vi "ziExample-Module-SweepUtility.vi"() -> ()   [LabVIEW 2009]
doc: "Control a Zurich instrument device via the LabOne Labview API. \nRequirements: Zurich Instruments MFLI, HF2 or UHFLI \nThis example shows how to start a sweeper module and retrieve data in an interactive vi.\n\n© Zurich Instruments AG, www.zhinst.com"
uses:
  <instrlib>/Zurich Instruments LabOne/Public/Modules/ziTypeModResults.ctl
  <instrlib>/Zurich Instruments LabOne/Public/Data/ziTypePollType.ctl
  <instrlib>/Zurich Instruments LabOne/Public/Modules/ziTypeModSWTriggerHeader.ctl
  <instrlib>/Zurich Instruments LabOne/Public/Modules/ziTypeModSweeperHeader.ctl
  <instrlib>/Zurich Instruments LabOne/Public/Modules/ziModSetValueBinary.vi
  <instrlib>/Zurich Instruments LabOne/Public/Modules/ziModGetDoubleData.vi
  <instrlib>/Zurich Instruments LabOne/Public/Modules/ziModGetSweeperData.vi
  <instrlib>/Zurich Instruments LabOne/Public/Modules/ziModSetValueDouble.vi
  <instrlib>/Zurich Instruments LabOne/Zurich Instruments LabOne.lvlib
panel:
  out "Error Out":errorcluster
  in  "Host:port (optional)":string
  out "Mod subs paths":string[](array[string])
  in  "demods/x/sample":bool[](array[boolean])
  in  "sweep/xmapping":i32(ring)=1 caption="X Mapping" items=["Linear", "Log"]
  in  "sweep/loopcount":i32=2 caption="Loop Count (#)" min=1 max=66000
  in  "sweep/order":u16(ring) caption="Order" items=["Current Setting", "6 dB/oct", "12 dB/oct", "18 dB/oct", "24 dB/oct", "30 dB/oct", "36 dB/oct", "42 dB/oct", "48 dB/oct"]
  out "Progress":dbl(slide) scale=0.0..1.0
  out "Finished?":bool
  out "sweep/remainingtime":dbl caption="Remaining Time (s)" format="%_5p"
  in  "sweep/settling/inaccuracy":dbl caption="Inaccuracy" format="%#_5p"
  in  "sweep/scan":u16(ring) caption="Scan" items=["Sequential", "Binary", "Bidirectional"]
  in  "sweep/settling/time":dbl caption="Settling (s)" format="%#_5p"
  in  "sweep/bandwidth":dbl caption="BW (Hz)" format="%#_5p"
  in  "sweep/bandwidthcontrol":u16(ring) caption="BW Control" items=["Manual", "Fixed", "Automatic"]
  in  "sweep/phaseunwrap":bool caption="Phase Unwrap"
  in  "sweep/maxbandwidth":dbl caption="Max BW (Hz)" format="%#_5p"
  in  "sweep/averaging/tc":dbl caption="Averaging TCs" format="%#_5p"
  in  "sweep/averaging/sample":dbl caption="Averaging Samples" format="%#_5p"
  in  "Stop Sweep":bool
  in  "sweep/endless":bool caption="Endless"
  in  "start_act":bool
  in  "sweepgridnode":string="oscs/0/freq" caption="sweep/gridnode"
  in  "sweep/omegasuppression":dbl caption="Omega Suppression (dB)" format="%#_5p"
  in  "sweep/sincfilter":bool caption="Sinc"
  in  "sweep/samplecount":i32=2 caption="Points (#)" min=2 max=66000
  in  "sweep/stop":dbl caption="Stop (Hz)" format="%_5p"
  in  "sweep/start":dbl caption="Start (Hz)" format="%_5p"
  in  "stop":bool
  in  "Address":string="DEV" caption="Device ID"
  out "Selected Device":string
  out "Sweeper Phase":cluster{"grid":dbl[], "phase":dbl[]}[](graph)
  out "Sweeper R":cluster{"grid":dbl[], "phase":dbl[]}[](graph)
  out "ziModResults":T1
  # "ziExample-SweepModul.vi\nRequirements: HF2LI, UHFLI or MFLI\nsee block diagram for VI description"
  # "Tested Devices:\n- MFLI\n- HF2LI\n- UHFLI"
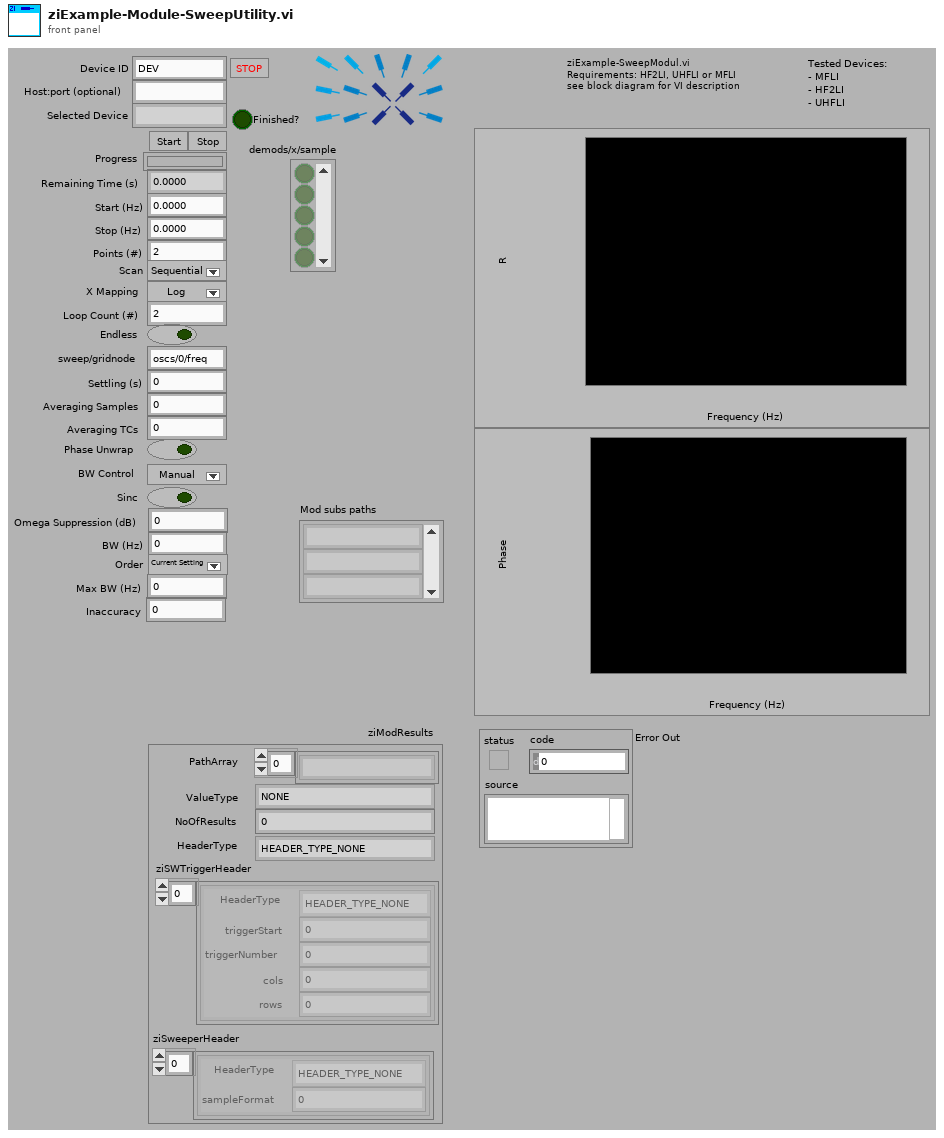
[diagram p1: front panel]
types:
  T1 = typedef "Zurich Instruments LabOne.lvlib/ziTypeModResults.ctl" = cluster{"PathArray":string[], "ValueType":T2, "NoOfResults":u64, "HeaderType":enum16{"HEADER_TYPE_NONE", "HEADER_TYPE_SWTRIGGER", "HEADER_TYPE_SWEEPER"}, "ziSWTriggerHeader":T3[], "ziSweeperHeader":T4[]}
  T2 = typedef "Zurich Instruments LabOne.lvlib/ziTypePollType.ctl" = enum16{"NONE", "DOUBLE_DATA", "INTEGER_DATA", "DEMOD_SAMPLE", "SCOPE_WAVE_HF2", "AUXIN_SAMPLE", "DIO_SAMPLE", "BYTE_ARRAY", "PWA_WAVE", "9", "10", "11", "12", "13", "14", "15", "TREE_CHANGE_DEPRI", "17", "ERROR", "19", "20", "21", "22", "23", "24", "25", "26", "27", "28", "29", "30", "31", "DOUBLE_DATA_TS", "INTEGER_DATA_TS", "34", "SCOPE_WAVE", "36", "37", "BYTE_ARRAY_TS", "39", "40", "41", "42", "43", "44", "45", "CNT_DATA", "47", "TREE_CHANGE", "49", "50", "51", "52", "53", "54", "55", "56", "57", "58", "59", "60", "61", "62", "63", "SWEEPER_DATA", "SPECTRUM_DATA", "ADVISOR_DATA", "67", "IMP_DATA"}
  T3 = typedef "Zurich Instruments LabOne.lvlib/ziTypeModSWTriggerHeader.ctl" = cluster{"HeaderType":enum8{"HEADER_TYPE_NONE", "HEADER_TYPE_SWTRIGGER", "HEADER_TYPE_SWEEPER"}, "triggerStart":u64, "triggerNumber":u64, "cols":u32, "rows":u32}
  T4 = typedef "Zurich Instruments LabOne.lvlib/ziTypeModSweeperHeader.ctl" = cluster{"HeaderType":enum8{"HEADER_TYPE_NONE", "HEADER_TYPE_SWTRIGGER", "HEADER_TYPE_SWEEPER"}, "sampleFormat":u8}
  T5 = typedef "Zurich Instruments LabOne.lvlib/ziTypeHandle.ctl" = cluster{"handleValid":bool, "Conn":u64, "Path Prefix":string, "Handle":u64, "Connected":bool, "Clockbase(s)":dbl}
  T6 = typedef "Zurich Instruments LabOne.lvlib/ziTypeModHandle.ctl" = cluster{"handleValid":bool, "Conn":u64, "ModHandle":u64, "moduleID":string, "Path Prefix":string}
  T7 = typedef "Zurich Instruments LabOne.lvlib/ziTypeModSweeperDemodWave.ctl" = cluster{"timestamp":u64, "sampleCount":u64, "flags":u8, "sampleFormat":u8, "sweepMode":u8, "bandwidthMode":u8, "count":u64[], "settimestamp":u64[], "nexttimestamp":u64[], "grid":dbl[], "bandwidth":dbl[], "tc":dbl[], "tcmeas":dbl[], "settling":dbl[], "x":dbl[], "xstddev":dbl[], "xpwr":dbl[], "y":dbl[], "ystddev":dbl[], "ypwr":dbl[], "r":dbl[], "rstddev":dbl[], "rpwr":dbl[], "phase":dbl[], "phasestddev":dbl[], "phasepwr":dbl[], "frequency":dbl[], "frequencystddev":dbl[], "frequencypwr":dbl[], "auxin0":dbl[], "auxin0stddev":dbl[], "auxin0pwr":dbl[], "auxin1":dbl[], "auxin1stddev":dbl[], "auxin1pwr":dbl[]}
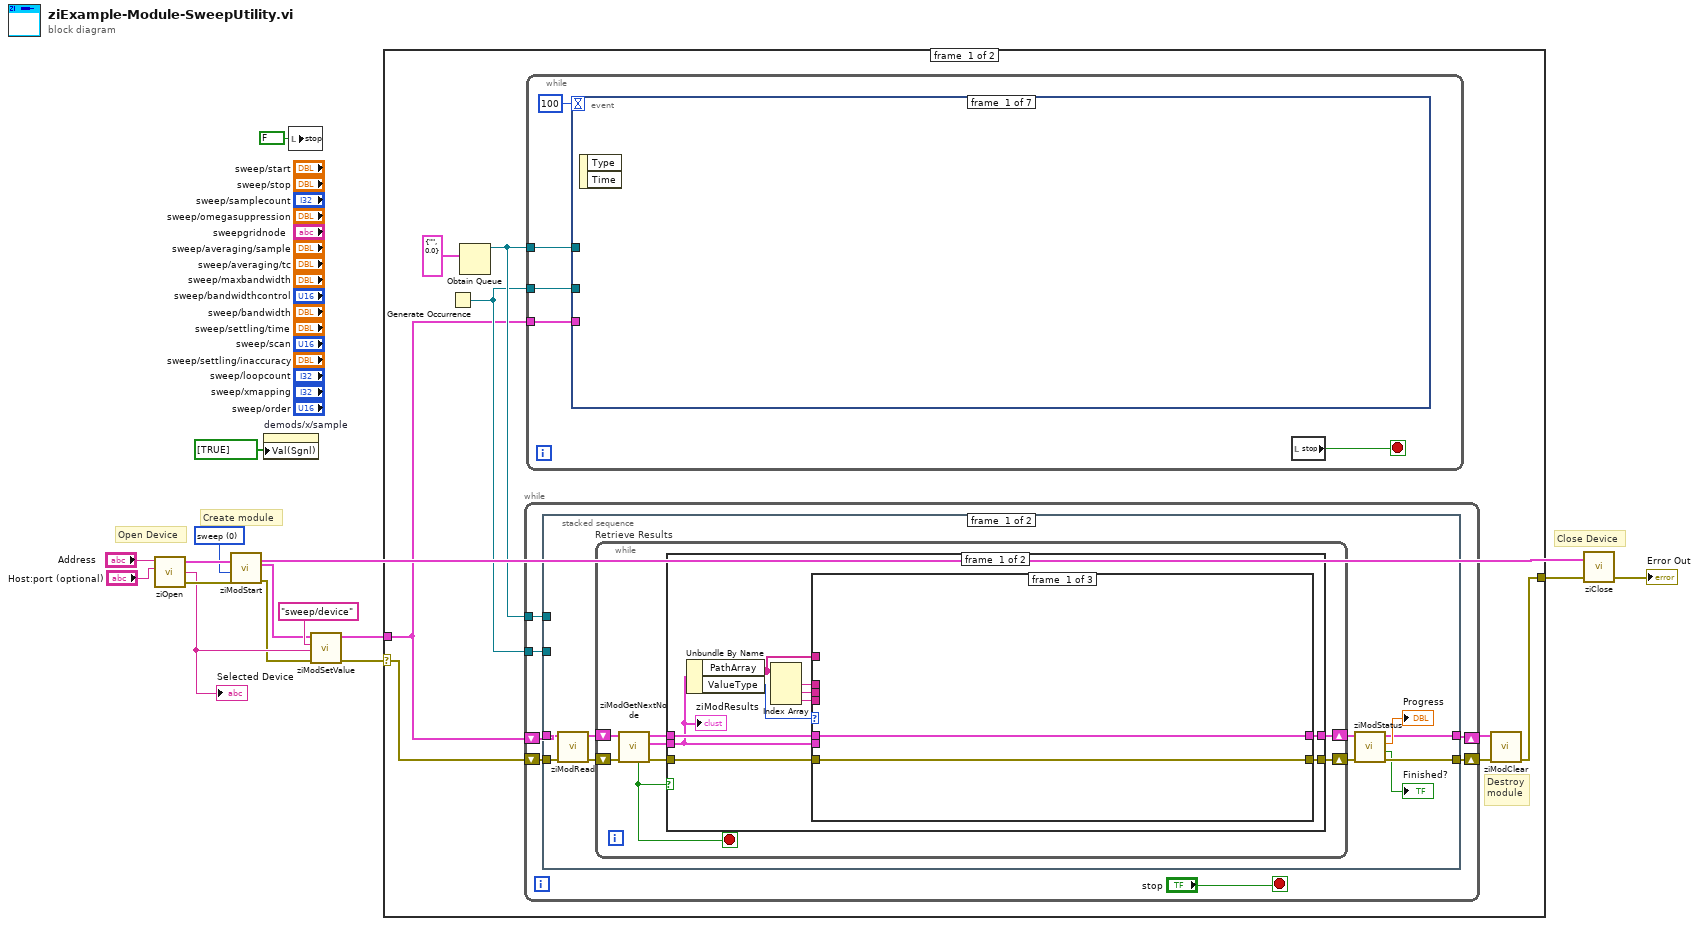
[diagram p0: block diagram]
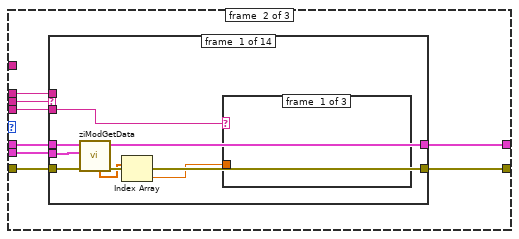
[diagram p2: hidden frame]
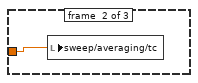
[diagram p3: hidden frame]
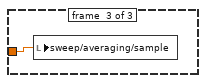
[diagram p4: hidden frame]
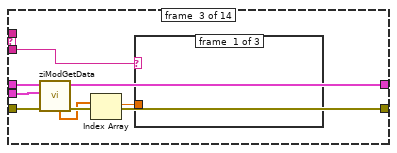
[diagram p6: hidden frame]
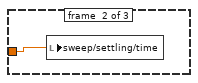
[diagram p7: hidden frame]
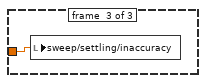
[diagram p8: hidden frame]
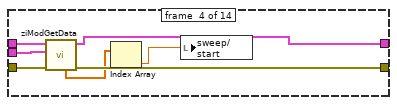
[diagram p9: hidden frame]
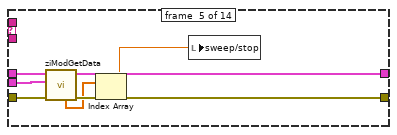
[diagram p10: hidden frame]
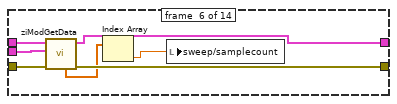
[diagram p11: hidden frame]
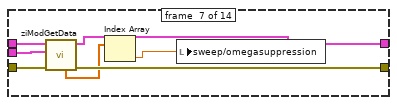
[diagram p12: hidden frame]
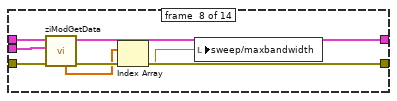
[diagram p13: hidden frame]
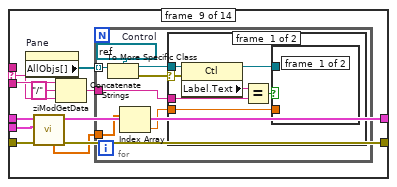
[diagram p14: hidden frame]
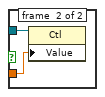
[diagram p15: hidden frame]
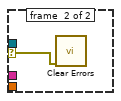
[diagram p16: hidden frame]
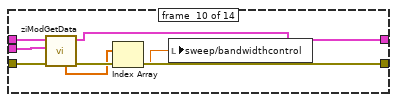
[diagram p17: hidden frame]
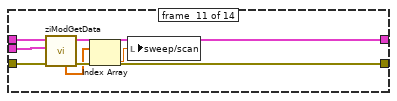
[diagram p18: hidden frame]
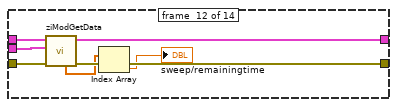
[diagram p19: hidden frame]
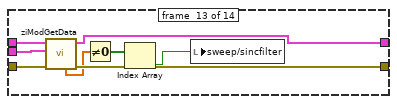
[diagram p20: hidden frame]
diagram:
  w11 = u16 0 items=["sweep", "zoomFFT", "deviceSettings", "record", "pllAdvisor", "pidAdvisor"] ("moduleID")
  # "Close Device"
  # "Create module"
  # "Open Device"
  n1 = call <instrlib>:"ziOpen.vi"("Hostname obsolete (auto)"="Host:port (optional)", "Address"="Address") -> ("Error Out"=w15:errorcluster, "Selected Device"=w14:string, "HandleOut"=w13:T5)  [unwired: 1 in, 1 out]
  "Selected Device" <- w14
  n2 = call <instrlib>:"ziModStart.vi"("Error In"=w15, "module Id"=w11, "Handle In"=w13) -> ("Error Out"=w10:errorcluster, "ModHandle Out"=w8:T6, "Handle Out"=w12:T5)  [unwired: 6 in]
  n3 = property on="demods/x/sample" class="Arr (strict)"("Val(Sgnl)"=bool[] [TRUE] ("Value (Signaling)")) -> ()  [unwired: 2 in, 2 out]
  n4 = local write "stop"(FALSE ("Stop")) -> ()
  n5 = call-poly <instrlib>:"ziModSetValue.vi"("Error In"=w10, "Data"=w14, "Path"="sweep/device", "ModHandle In"=w8) -> ("Error Out"=w5:errorcluster, "ModHandle Out"=w7:T6)  [unwired: 6 in]
  n6 = case shown="No Error" w5 {
    selector: w5 -> [w17 w317]
    tunnel: [w24 w317] -> w16
    tunnel: w7 -> [w18 _]
    frame #0 {
      # "Destroy\nmodule"
      n7 = Generate Occurrence() -> (w19:refnum<k4>)
      n8 = Obtain Queue(element data type=cluster{"Label.Text":string, "sweep/stop":dbl} {"Label.Text"="", "sweep/stop"=0.0} ("output cluster")) -> (queue out=w20:refnum<queue>)  [unwired: 4 in, 2 out]
      n9 = while {
        shift-right: [w27] -> w23
        shift-left: w18 -> [w30]
        shift-right: [w31] -> w22
        shift-left: w17 -> [w29]
        tunnel: w20 -> [w26]
        tunnel: w19 -> [w25]
        stop <- "stop" stop-if-true
        n10 = stacked-sequence {
          tunnel: [w33 _] -> w31
          tunnel: w30 -> [w41 w245]
          tunnel: w29 -> [w40 _]
          tunnel: [w35 _] -> w27
          tunnel: w26 -> [_ w246]
          tunnel: w25 -> [_ w243]
          frame #0 {
            n11 = call <instrlib>:"ziModRead.vi"("error in"=w40, "ziModHandle In"=w41) -> ("error out"=w39:errorcluster, "ziModHandle Out"=w38:T6)  [unwired: 8 in]
            n12 = while "Retrieve Results" {
              shift-right: [w46] -> w37
              shift-left: w38 -> [w48]
              shift-right: [w45] -> w34
              shift-left: w39 -> [w49]
              stop <- w42 stop-if-true
              n13 = call <instrlib>:"ziModGetNextNode.vi"("Error In"=w49, "ModHandle In"=w48) -> ("Error Out"=w43:errorcluster, "ModResults"=w44:T1, "ModHandle Out"=w47:T6, "NoData"=w42:bool)  [unwired: 6 in]
              n14 = case shown="False" w42 {
                tunnel: w47 -> [w59 w236]
                tunnel: [w56 w236] -> w46
                tunnel: [w55 w237] -> w45
                tunnel: w44 -> [w52 _]
                tunnel: w43 -> [w50 w237]
                frame #0 {
                  n15 = Unbundle By Name(w52) -> ("PathArray"=w51:string[], "ValueType"=w54:T2)
                  n16 = Index Array(array=w51) -> (element #1=w53:string, element #2=w58:string, element #3=w57:string)  [unwired: 3 in]
                  n17 = case shown="\"SWEEPER_DATA\"" w54 {
                    tunnel: w59 -> [w61 w69 w223]
                    tunnel: w52 -> [_ w68 w203]
                    tunnel: w50 -> [w60 w67 w222]
                    tunnel: w58 -> [_ w66 _]
                    tunnel: w57 -> [_ w65 w219]
                    tunnel: [w61 w64 w220] -> w56
                    tunnel: [w60 w63 w221] -> w55
                    tunnel: w53 -> [_ w62 _]
                    tunnel: w51 -> [_ _ w194]
                    frame #0 {
                    }
                    frame #1 {
                      n18 = case shown="\"endless\"" w66 {
                        selector: w66 -> [_ _ _ _ _ _ _ _ w130 _ _ _ _ _]
                        tunnel: w69 -> [w74 w81 w86 w98 w105 w112 w119 w126 w137 w161 w168 w175 w183 w191]
                        tunnel: w68 -> [w75 _ w87 w94 w101 w108 w116 w122 w133 w157 w164 w171 w179 w187]
                        tunnel: w67 -> [w76 w80 w88 w95 w102 w109 w117 w123 w134 w158 w165 w172 w180 w188]
                        tunnel: [w72 w80 w84 w96 w103 w110 w115 w124 w135 w159 w166 w173 w181 w189] -> w63
                        tunnel: [w73 w81 w85 w97 w104 w111 w118 w125 w136 w160 w167 w174 w182 w190] -> w64
                        tunnel: w65 -> [w77 _ w89 _ _ _ _ _ _ _ _ _ _ _]
                        tunnel: w62 -> [_ _ _ _ _ _ _ _ w131 _ _ _ _ _]
                        frame #0 {
                          n19 = call-poly <instrlib>:"ziModGetData.vi"("Error In"=w76, "ModResults"=w75, "ModHandle In"=w74) -> ("Error Out"=w72:errorcluster, "ModHandle Out"=w73:T6, "Value"=w70:dbl[])  [unwired: 4 in, 2 out]
                          n20 = Index Array(array=w70) -> (element=w71:dbl)  [unwired: 1 in]
                          n21 = case shown="\"sample\"" w77 {
                            tunnel: w71 -> [_ w78 w79]
                            frame #0 {
                            }
                            frame #1 {
                              n22 = local write "sweep/averaging/tc"(w78) -> ()
                            }
                            frame #2 {
                              n23 = local write "sweep/averaging/sample"(w79) -> ()
                            }
                          }
                        }
                        frame #1 {
                        }
                        frame #2 {
                          n24 = call-poly <instrlib>:"ziModGetData.vi"("Error In"=w88, "ModResults"=w87, "ModHandle In"=w86) -> ("Error Out"=w84:errorcluster, "ModHandle Out"=w85:T6, "Value"=w82:dbl[])  [unwired: 4 in, 2 out]
                          n25 = Index Array(array=w82) -> (element=w83:dbl)  [unwired: 1 in]
                          n26 = case shown="\"time\"" w89 {
                            tunnel: w83 -> [_ w90 w91]
                            frame #0 {
                            }
                            frame #1 {
                              n27 = local write "sweep/settling/time"(w90) -> ()
                            }
                            frame #2 {
                              n28 = local write "sweep/settling/inaccuracy"(w91) -> ()
                            }
                          }
                        }
                        frame #3 {
                          n29 = call-poly <instrlib>:"ziModGetData.vi"("Error In"=w95, "ModResults"=w94, "ModHandle In"=w98) -> ("Error Out"=w96:errorcluster, "ModHandle Out"=w97:T6, "Value"=w93:dbl[])  [unwired: 4 in, 2 out]
                          n30 = Index Array(array=w93) -> (element=w92:dbl)  [unwired: 1 in]
                          n31 = local write "sweep/start"(w92) -> ()
                        }
                        frame #4 {
                          n32 = call-poly <instrlib>:"ziModGetData.vi"("Error In"=w102, "ModResults"=w101, "ModHandle In"=w105) -> ("Error Out"=w103:errorcluster, "ModHandle Out"=w104:T6, "Value"=w99:dbl[])  [unwired: 4 in, 2 out]
                          n33 = Index Array(array=w99) -> (element=w100:dbl)  [unwired: 1 in]
                          n34 = local write "sweep/stop"(w100) -> ()
                        }
                        frame #5 {
                          n35 = call-poly <instrlib>:"ziModGetData.vi"("Error In"=w109, "ModResults"=w108, "ModHandle In"=w112) -> ("Error Out"=w110:errorcluster, "ModHandle Out"=w111:T6, "Value"=w107:dbl[])  [unwired: 4 in, 2 out]
                          n36 = Index Array(array=w107) -> (element=w106:dbl)  [unwired: 1 in]
                          n37 = local write "sweep/samplecount"(w106) -> ()
                        }
                        frame #6 {
                          n38 = call-poly <instrlib>:"ziModGetData.vi"("Error In"=w117, "ModResults"=w116, "ModHandle In"=w119) -> ("Error Out"=w115:errorcluster, "ModHandle Out"=w118:T6, "Value"=w114:dbl[])  [unwired: 4 in, 2 out]
                          n39 = Index Array(array=w114) -> (element=w113:dbl)  [unwired: 1 in]
                          n40 = local write "sweep/omegasuppression"(w113) -> ()
                        }
                        frame #7 {
                          n41 = call-poly <instrlib>:"ziModGetData.vi"("Error In"=w123, "ModResults"=w122, "ModHandle In"=w126) -> ("Error Out"=w124:errorcluster, "ModHandle Out"=w125:T6, "Value"=w121:dbl[])  [unwired: 4 in, 2 out]
                          n42 = Index Array(array=w121) -> (element=w120:dbl)  [unwired: 1 in]
                          n43 = local write "sweep/maxbandwidth"(w120) -> ()
                        }
                        frame #8 {
                          n44 = property on="Pane" class="Pane"() -> ("AllObjs[]"=w132:refnum<vi>[])  [unwired: 2 in, 2 out]
                          n45 = call-poly <instrlib>:"ziModGetData.vi"("Error In"=w134, "ModResults"=w133, "ModHandle In"=w137) -> ("Error Out"=w135:errorcluster, "ModHandle Out"=w136:T6, "Value"=w127:dbl[])  [unwired: 4 in, 2 out]
                          n46 = Concatenate Strings(w131, "/" ("string"), w130) -> (w128:string)
                          n47 = for {
                            tunnel: w132 -> [w142] mode=indexing
                            tunnel: w128 -> [w141]
                            tunnel: w127 -> [w138]
                            w144 = refnum<vi> refnum  # Control
                            n48 = To More Specific Class(target class=w144, reference=w142) -> (specific class reference=w143:refnum<vi>, error out=w140:errorcluster)  [unwired: 1 in]
                            n49 = Index Array(array=w138) -> (element=w139:dbl)  [unwired: 1 in]
                            n50 = case shown="No Error" w140 {
                              selector: w140 -> [w145 w154]
                              tunnel: w143 -> [w151 _]
                              tunnel: w141 -> [w149 _]
                              tunnel: w139 -> [w146 _]
                              frame #0 {
                                n51 = property class="Ctl"(reference=w151, error in=w145) -> (reference out=w147:refnum<vi>, "Label.Text"=w150:string)  [unwired: 1 out]
                                n52 = Equal?(x=w150, y=w149) -> (x = y?=w148:bool)
                                n53 = case shown="True" w148 {
                                tunnel: w147 -> [_ w153]
                                tunnel: w146 -> [_ w152]
                                frame #0 {
                                }
                                frame #1 {
                                n54 = property class="Ctl"(reference=w153, "Value"=w152) -> ()  [unwired: 1 in, 2 out]
                                }
                                }
                              }
                              frame #1 {
                                n55 = call <vilib>:"Clear Errors.vi"("error in (no error)"=w154) -> ()  [unwired: 6 in, 1 out]
                              }
                            }
                          }
                        }
                        frame #9 {
                          n56 = call-poly <instrlib>:"ziModGetData.vi"("Error In"=w158, "ModResults"=w157, "ModHandle In"=w161) -> ("Error Out"=w159:errorcluster, "ModHandle Out"=w160:T6, "Value"=w156:dbl[])  [unwired: 4 in, 2 out]
                          n57 = Index Array(array=w156) -> (element=w155:dbl)  [unwired: 1 in]
                          n58 = local write "sweep/bandwidthcontrol"(w155) -> ()
                        }
                        frame #10 {
                          n59 = call-poly <instrlib>:"ziModGetData.vi"("Error In"=w165, "ModResults"=w164, "ModHandle In"=w168) -> ("Error Out"=w166:errorcluster, "ModHandle Out"=w167:T6, "Value"=w163:dbl[])  [unwired: 4 in, 2 out]
                          n60 = Index Array(array=w163) -> (element=w162:dbl)  [unwired: 1 in]
                          n61 = local write "sweep/scan"(w162) -> ()
                        }
                        frame #11 {
                          n62 = call-poly <instrlib>:"ziModGetData.vi"("Error In"=w172, "ModResults"=w171, "ModHandle In"=w175) -> ("Error Out"=w173:errorcluster, "ModHandle Out"=w174:T6, "Value"=w170:dbl[])  [unwired: 4 in, 2 out]
                          n63 = Index Array(array=w170) -> (element=→"sweep/remainingtime":dbl)  [unwired: 1 in]
                        }
                        frame #12 {
                          n64 = call-poly <instrlib>:"ziModGetData.vi"("Error In"=w180, "ModResults"=w179, "ModHandle In"=w183) -> ("Error Out"=w181:errorcluster, "ModHandle Out"=w182:T6, "Value"=w177:dbl[])  [unwired: 4 in, 2 out]
                          n65 = Not Equal To 0?(x=w177) -> (x != 0?=w178:bool[])
                          n66 = Index Array(array=w178) -> (element=w176:bool)  [unwired: 1 in]
                          n67 = local write "sweep/sincfilter"(w176) -> ()
                        }
                        frame #13 {
                          n68 = call-poly <instrlib>:"ziModGetData.vi"("Error In"=w188, "ModResults"=w187, "ModHandle In"=w191) -> ("Error Out"=w189:errorcluster, "ModHandle Out"=w190:T6, "Value"=w185:dbl[])  [unwired: 4 in, 2 out]
                          n69 = Not Equal To 0?(x=w185) -> (x != 0?=w186:bool[])
                          n70 = Index Array(array=w186) -> (element=w184:bool)  [unwired: 1 in]
                          n71 = local write "sweep/endless"(w184) -> ()
                        }
                      }
                    }
                    frame #2 {
                      n72 = call-poly <instrlib>:"ziModGetData.vi"("Error In"=w222, "ModResults"=w203, "ModHandle In"=w223) -> ("Error Out"=w221:errorcluster, "SweeperDemodWaveArray"=w206:T7[], "ModHandle Out"=w220:T6)  [unwired: 4 in, 2 out]
                      n73 = local read "Mod subs paths"() -> (w196:string[])
                      n74 = Delete From Array(array=w194, length=3 ("index"), index=0) -> (array with subset deleted=w193:string[])  [unwired: 1 out]
                      n75 = Reverse 1D Array(array=w206) -> (reversed array=w205:T7[])
                      n76 = for {
                        tunnel: w193 -> [w234] mode=indexing
                        shift-right: [w233] -> w199
                        shift-left: w219 -> [w232]
                        n77 = Concatenate Strings(w232, "/" ("string"), w234) -> (w233:string)
                      }
                      n78 = Index Array(array=w205) -> (element=w215:T7)  [unwired: 1 in]
                      n79 = To Lower Case(string=w196) -> (all lower case string=w195:string[])
                      n80 = Unbundle By Name(w215) -> ("grid"=w216:dbl[], "r"=w218:dbl[], "phase"=w217:dbl[])
                      n81 = Bundle("grid"=w216, "phase"=w217) -> (w204:cluster{"grid":dbl[], "phase":dbl[]})  [unwired: 1 in]
                      n82 = Bundle("grid"=w216, "r"=w218) -> (w211:cluster{"grid":dbl[], "r":dbl[]})  [unwired: 1 in]
                      n83 = Search 1D Array(1D array=w195, element=w199) -> (index of element=w198:i32)  [unwired: 1 in]
                      n84 = Array Size(array=w195) -> (size(s)=w212:i32)
                      n85 = Build Array(w211, w204) -> (w202:cluster{"grid":dbl[], "phase":dbl[]}[])
                      n86 = Array Size(array=w202) -> (size(s)=w201:i32)
                      n87 = feedback #1(cluster{"grid":dbl[], "phase":dbl[]}[][] []) -> (w210:cluster{"grid":dbl[], "phase":dbl[]}[][])
                      n88 = case shown="Default" w198 {
                        selector: w198 -> [_ w225]
                        tunnel: w212 -> [_ w231]
                        tunnel: w210 -> [w224 w229]
                        tunnel: [w224 w228] -> w209
                        tunnel: w202 -> [_ w227]
                        tunnel: w201 -> [_ w226]
                        frame #0 {
                        }
                        frame #1 {
                          n89 = Reshape Array(w229, w231, w226) -> (w230:cluster{"grid":dbl[], "phase":dbl[]}[][])
                          n90 = Replace Array Subset(array=w230, new element=w227, index (row)=w225) -> (w228:cluster{"grid":dbl[], "phase":dbl[]}[][])  [unwired: 1 in]
                        }
                      }
                      n91 = Index Array(array=w209, index (col) #1=0 ("disabled index (col)"), index (col) #2=1 ("index (col)")) -> (element #1=→"Sweeper R":cluster{"grid":dbl[], "phase":dbl[]}[], element #2=→"Sweeper Phase":cluster{"grid":dbl[], "phase":dbl[]}[])  [unwired: 2 in]
                    }
                  }
                  "ziModResults" <- w52
                }
                frame #1 {
                  n92 = Wait (ms)(milliseconds to wait=u32 50) -> ()  [unwired: 1 out]
                }
              }
            }
            n93 = call <instrlib>:"ziModStatus.vi"("Error In"=w34, "ModHandle IN"=w37) -> ("Error Out"=w33:errorcluster, "Finished?"=→"Finished?":bool, "Progress (unity)"=→"Progress":dbl, "ModHandle Out"=w35:T6)  [unwired: 5 in]
          }
          frame #1 {
            n94 = Flush Queue(queue=w246) -> (remaining elements=w244:cluster{"Label.Text":string, "sweep/stop":dbl}[])  [unwired: 1 in, 2 out]
            n95 = Wait on Occurrence(1:FALSE ("ignore previous (T)"), 2:w243, 3:0 ("ms timeout (-1)")) -> (0:w241:bool)
            n96 = for {
              tunnel: w244 -> [w254] mode=indexing
              shift-right: [w253] -> w240
              shift-left: w245 -> [w255]
              n97 = Unbundle(w254) -> ("Label.Text"=w256:string, "sweep/stop"=w252:dbl)
              n98 = call-poly <instrlib>:"ziModSetValue.vi"("Value"=w252, "Path"=w256, "ModHandle In"=w255) -> ("ModHandle Out"=w253:T6)  [unwired: 7 in, 1 out]
            }
            n99 = case shown="False" w241 {
              tunnel: w240 -> [w249 w251]
              tunnel: [w248 w251] -> _
              frame #0 {
                n100 = call <instrlib>:"ziModExecute.vi"("Modal (F)"=TRUE ("Modal"), "ziModHandle In"=w249) -> ("ziModHandle Out"=w248:T6)  [unwired: 6 in, 2 out]
                n101 = property on="start_act" class="Bool (strict)"("Value"=FALSE) -> ()  [unwired: 2 in, 2 out]
              }
              frame #1 {
              }
            }
          }
        }
      }
      n102 = while {
        tunnel: w18 -> [w261]
        tunnel: w20 -> [w258]
        tunnel: w19 -> [w257]
        stop <- w260 stop-if-true
        n103 = event shown="[6] \"Stop Sweep\": Value Change" {
          selector: _ -> [_ _ _ _ _ _ _]
          dyn-events: _ -> [_ _ _ _ _ _ _]
          timeout: 100 -> [_ _ _ _ _ _ _]
          tunnel: w261 -> [_ w269 w278 w289 w294 w299 w316]
          tunnel: w258 -> [_ w265 w273 _ _ _ _]
          tunnel: w257 -> [_ _ _ _ w293 _ _]
          event #0 {
            n104 = event-data() -> ()  [unwired: 1 in, 2 out]
          }
          event #1 {
            n105 = event-data() -> ("CtlRef"=w266:refnum<vi>, "NewVal"=w267:variant)  [unwired: 1 in, 3 out]
            n106 = property class="Num"(reference=w266) -> ("Label.Text"=w264:string)  [unwired: 1 in, 2 out]
            n107 = Variant To Data(Variant=w267, type=0.0 ("sweep/stop")) -> (data=w263:dbl)  [unwired: 1 in, 1 out]
            n108 = Bundle("Label.Text"=w264, "sweep/stop"=w263) -> (w262:cluster{"Label.Text":string, "sweep/stop":dbl})  [unwired: 1 in]
            n109 = Enqueue Element(queue=w265, element=w262) -> ()  [unwired: 2 in, 3 out]
            n110 = disable-structure shown="Enabled" {
              disable-tunnel: w269 -> [w272 _]
              disable-tunnel: w264 -> [w271 _]
              disable-tunnel: w263 -> [w270 _]
              frame #0 {
                n111 = call-poly <instrlib>:"ziModSetValue.vi"("Value"=w270, "Path"=w271, "ModHandle In"=w272) -> ()  [unwired: 2 in, 2 out]
              }
              frame #1 {
              }
            }
          }
          event #2 {
            n112 = event-data() -> ("CtlRef"=w277:refnum<vi>, "NewVal"=w274:bool)  [unwired: 1 in, 3 out]
            n113 = property class="Bool (strict)"(reference=w277) -> ("Label.Text"=w276:string)  [unwired: 1 in, 2 out]
            n114 = Boolean To (0,1)(Boolean=w274) -> (0, 1=w275:i16)
            n115 = disable-structure shown="Enabled" {
              disable-tunnel: w278 -> [w281 _]
              disable-tunnel: w276 -> [w280 w284]
              disable-tunnel: w275 -> [w279 w283]
              disable-tunnel: w273 -> [_ w282]
              frame #0 {
                n116 = call-poly <instrlib>:"ziModSetValue.vi"("Value"=w279, "Path"=w280, "ModHandle In"=w281) -> ()  [unwired: 2 in, 2 out]
              }
              frame #1 {
                n117 = Bundle("Label.Text"=w284, w283) -> (w285:cluster{"Label.Text":string, i16})  [unwired: 1 in]
                n118 = Enqueue Element(queue=w282, element=w285) -> ()  [unwired: 2 in, 3 out]
              }
            }
          }
          event #3 {
            n119 = event-data() -> ("CtlRef"=w288:refnum<vi>, "NewVal"=w286:string)  [unwired: 1 in, 3 out]
            n120 = property class="Str"(reference=w288) -> ("Label.Text"=w287:string)  [unwired: 1 in, 2 out]
            n121 = disable-structure shown="Disabled" {
              disable-tunnel: w289 -> [w292 _]
              disable-tunnel: w287 -> [w291 _]
              disable-tunnel: w286 -> [w290 _]
              frame #0 {
                n122 = call-poly <instrlib>:"ziModSetValue.vi"("Data"=w290, "Path"=w291, "ModHandle In"=w292) -> ()  [unwired: 2 in, 2 out]
              }
              frame #1 {
              }
            }
          }
          event #4 {
            n123 = event-data() -> ()  [unwired: 1 in, 5 out]
            n124 = Set Occurrence(w293) -> ()
            n125 = disable-structure shown="Disabled" {
              disable-tunnel: w294 -> [w295 _]
              frame #0 {
                n126 = call <instrlib>:"ziModExecute.vi"("Modal (F)"=TRUE ("Modal"), "ziModHandle In"=w295) -> ()  [unwired: 6 in, 3 out]
              }
              frame #1 {
              }
            }
          }
          event #5 {
            n127 = event-data() -> ()  [unwired: 1 in, 5 out]
            n128 = for {
              tunnel: "demods/x/sample" -> [w308] mode=indexing
              tunnel: "demods/%d/sample" -> [w305]
              tunnel: w299 -> [w307]
              shift-right: [w302] -> w297
              shift-left: string[] [] ("Mod subs paths") -> [w304]
              i -> [w306]
              n129 = Format Into String(format string=w305, w306) -> (resulting string=w303:string)  [unwired: 2 in, 1 out]
              n130 = case shown="True" w308 {
                tunnel: w307 -> [w311 w315]
                tunnel: w304 -> [w309 w314]
                tunnel: w303 -> [w310 w313]
                tunnel: [w309 w312] -> w302
                frame #0 {
                  n131 = call <instrlib>:"ziModUnSubscribe.vi"("Path (\"/\")"=w310, "ModHandle In"=w311) -> ()  [unwired: 8 in, 2 out]
                }
                frame #1 {
                  n132 = call <instrlib>:"ziModSubscribe.vi"("Path"=w313, "ModHandle In"=w315) -> ()  [unwired: 7 in, 2 out]
                  n133 = Build Array (concatenate)(w314, w313) -> (w312:string[])
                }
              }
            }
            "Mod subs paths" <- w297
          }
          event #6 {
            n134 = event-data() -> ()  [unwired: 1 in, 5 out]
            n135 = call <instrlib>:"ziModFinish.vi"("ziModHandle In"=w316) -> ()  [unwired: 8 in, 2 out]
          }
        }
        n136 = local read "stop"() -> (w260:bool)
      }
      n137 = call <instrlib>:"ziModClear.vi"("Error In"=w22, "ziModHandle In"=w23) -> ("Error Out"=w24:errorcluster)  [unwired: 7 in, 1 out]
    }
    frame #1 {
    }
  }
  n138 = call <instrlib>:"ziClose.vi"("Error In"=w16, "Handle In"=w12) -> ("Error Out"=→"Error Out":errorcluster)  [unwired: 2 in, 1 out]
